vi "Auto Fit and Save Calibration Curve_YCC.vi"() -> ()   [LabVIEW 2014]
uses:
  <vilib>/Utility/file.llb/Write To Spreadsheet File (DBL).vi
  <vilib>/Utility/file.llb/Read From Spreadsheet File (DBL).vi
  <vilib>/Analysis/NI_AALPro.lvlib
  <vilib>/gmath/NI_Gmath.lvlib
panel:
  in  "defalut save?":bool=TRUE
  in  "X=T\nY=F":bool=TRUE
  out "save to path":path
  out "Polynomial Coefficients":dbl[](array[numeric])
  out "r^2":dbl format="%.7g"
  out "correlation coefficient r":dbl format="%.7g"
  out "folder exists?":bool
  in  "Save to Calibration File?":bool
  in  "Tab Control":enum32{"Sensitivity Fit", "Stiffness Fit"}(tab)
  in  "Folder Path":path
  out "Number of Files":i32
  in  "radius range wanted to fit (nm)":dbl=100.0
  out "All slope":dbl[](array[numeric])
  out "abs (All slope )":dbl[](array[numeric])
  out "XY Graph":cluster{dbl[], "abs (All slope )":dbl[]}[](graph)
  out "All laserpower (mW)":dbl[](array[numeric])
  out "Path":path
  in  "match substring":string="-Stuckbead Scan-"
  out "XY Graph 2":cluster{"all rows":dbl[], "all rows":dbl[]}[](graph)
  in  "file path (dialog if empty)":path
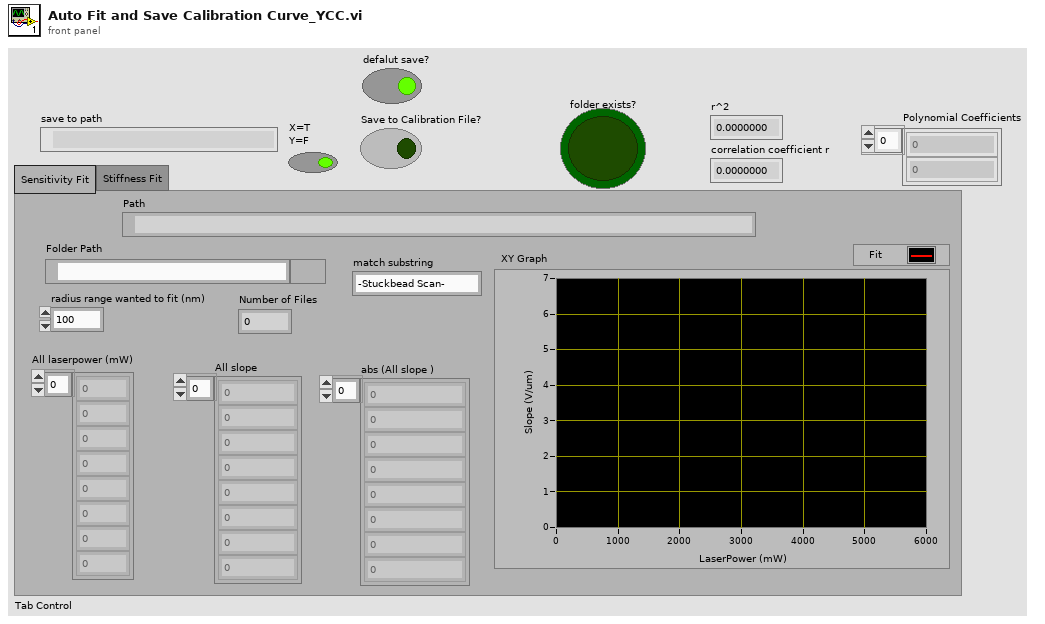
[diagram p1: front panel]
types:
  T1 = cluster{"All laserpower (mW)":dbl[], "Best Polynomial Fit":dbl[]}
  T2 = cluster{"All laserpower (mW)":dbl[], "abs (All slope )":dbl[]}
  T3 = cluster{"All laserpower (mW)":dbl[], "abs (All slope )":dbl[]}[]
  T4 = cluster{"all rows":dbl[], "Best Polynomial Fit":dbl[]}
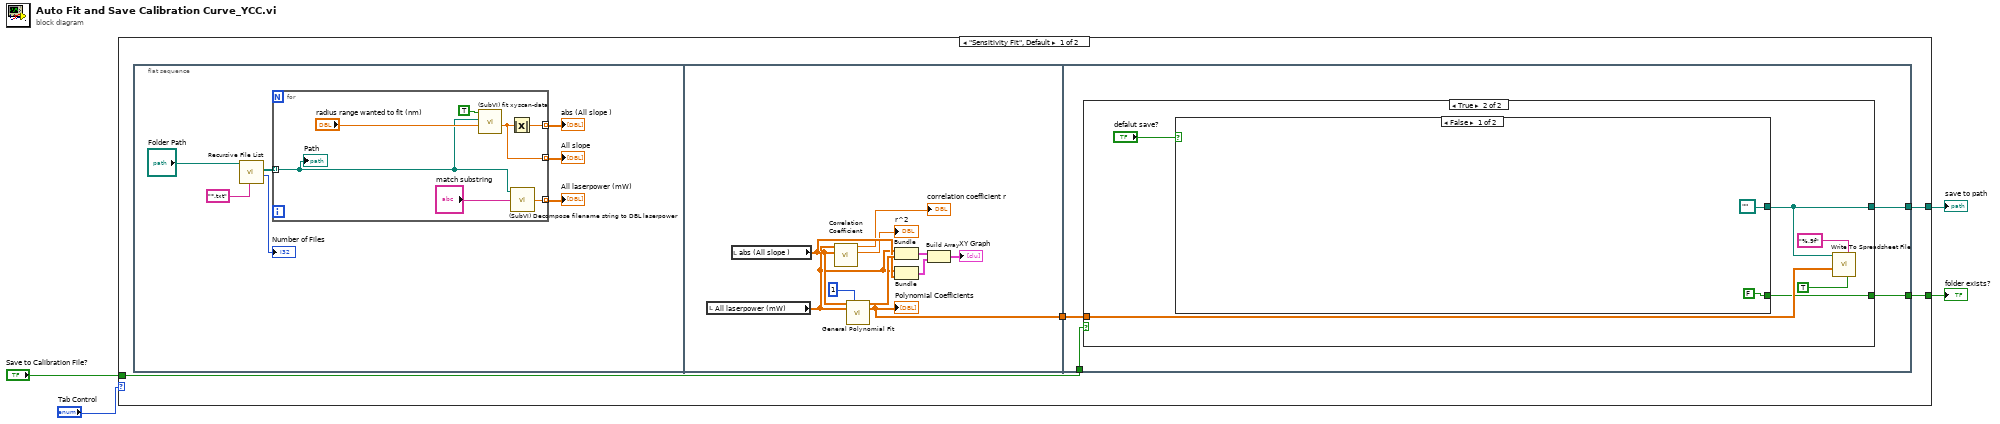
[diagram p0: block diagram]
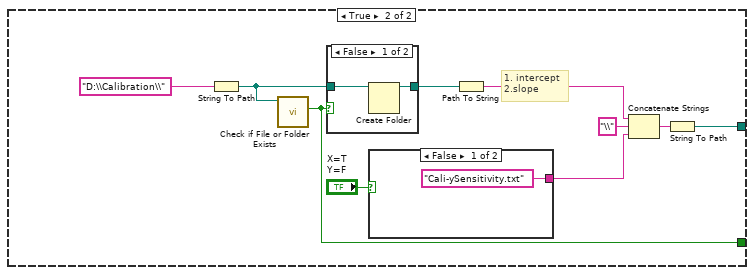
[diagram p3: hidden frame]
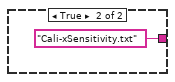
[diagram p4: hidden frame]
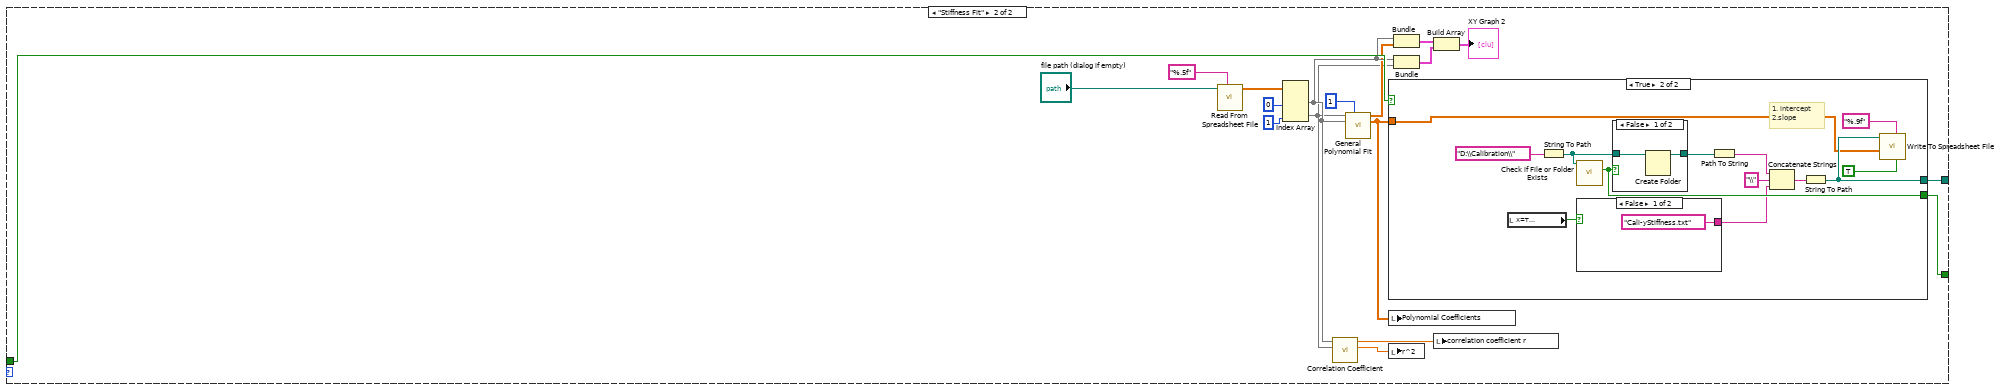
[diagram p6: hidden frame]
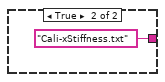
[diagram p8: hidden frame]
diagram:
  n1 = case shown="\"Sensitivity Fit\", Default" "Tab Control" {
    tunnel: "Save to Calibration File?" -> [w7 w77]
    tunnel: [w6 w75] -> w2
    tunnel: [w5 w76] -> w1
    frame "Sensitivity Fit", Default {
      n2 = flat-sequence {
        tunnel: [w24] -> w8
        tunnel: w8 -> [w36]
        tunnel: w7 -> [w35]
        tunnel: [w34] -> w6
        tunnel: [w33] -> w5
        frame #0 {
          n3 = call <vilib>:"Recursive File List.vi"("pattern"="*.txt", "Folder Path"="Folder Path") -> ("Number of Files"=→"Number of Files":i32, "All Files in Dir"=w12:path[])  [unwired: 5 in, 3 out]
          n4 = for {
            tunnel: w12 -> [w18] mode=indexing
            tunnel: [w20] -> w11 mode=indexing
            tunnel: [w19] -> w10 mode=indexing
            tunnel: [w17] -> w9 mode=indexing
            n5 = call "(SubVI) fit xyscan-data.vi"("range wanted to fit"="radius range wanted to fit (nm)", "file path (dialog if empty)"=w18, "X=T\nY=F"=TRUE ("X=T\nY=F")) -> ("Slope (V/um)"=w20:dbl)  [unwired: 4 in]
            n6 = Absolute Value(x=w20) -> (abs(x)=w19:dbl)
            n7 = call "(SubVI) Decompose filename string to DBL laserpower.vi"("match substring"="match substring", "path"=w18) -> ("LaserPower (mW)"=w17:dbl)  [unwired: 3 in]
            "Path" <- w18
          }
          "All slope" <- w11
          "abs (All slope )" <- w10
          "All laserpower (mW)" <- w9
        }
        frame #1 {
          n8 = local read "All laserpower (mW)"() -> (w23:dbl[])
          n9 = local read "abs (All slope )"() -> (w27:dbl[])
          n10 = call <vilib>:"Correlation Coefficient.vi"("Y"=w27, "X"=w23) -> ("r^2"=→"r^2":dbl, "correlation coefficient r"=→"correlation coefficient r":dbl)  [unwired: 8 in]
          n11 = call <vilib>:"General Polynomial Fit.vi"("Y"=w27, "polynomial order"=1, "X"=w23) -> ("Best Polynomial Fit"=w32:dbl[], "Polynomial Coefficients"=w24:dbl[])  [unwired: 9 in, 2 out]
          "Polynomial Coefficients" <- w24
          n12 = Bundle("All laserpower (mW)"=w23, "Best Polynomial Fit"=w32) -> (w31:T1)  [unwired: 1 in]
          n13 = Bundle("All laserpower (mW)"=w23, "abs (All slope )"=w27) -> (w30:T2)  [unwired: 1 in]
          n14 = Build Array(w31, w30) -> (→"XY Graph":T3)
        }
        frame #2 {
          n15 = case shown="True" w35 {
            tunnel: w36 -> [_ w42]
            tunnel: [_ w39] -> w34
            tunnel: [_ w38] -> w33
            frame False {
            }
            frame True {
              n16 = case shown="False" "defalut save?" {
                tunnel: [path "" w47] -> w39
                tunnel: [FALSE ("file or folder exists?") w46] -> w38
                frame False {
                }
                frame True {
                  # "1. intercept\n2.slope"
                  n17 = String To Path(string="D:\\Calibration\\") -> (path=w54:path)
                  n18 = call <vilib>:"Check if File or Folder Exists.vi"("path"=w54) -> ("file or folder exists?"=w46:bool)  [unwired: 8 in, 2 out]
                  n19 = case shown="False" w46 {
                    tunnel: w54 -> [w58 w59]
                    tunnel: [w57 w59] -> w52
                    frame False {
                      n20 = Create Folder(path (use dialog)=w58) -> (created path=w57:path)  [unwired: 2 in, 2 out]
                    }
                    frame True {
                    }
                  }
                  n21 = case shown="False" "X=T\nY=F" {
                    tunnel: ["Cali-ySensitivity.txt" "Cali-xSensitivity.txt"] -> w49
                    frame False {
                    }
                    frame True {
                    }
                  }
                  n22 = Path To String(path=w52) -> (string=w51:string)
                  n23 = Concatenate Strings(w51, "\\", w49) -> (w50:string)
                  n24 = String To Path(string=w50) -> (path=w47:path)
                }
              }
              n25 = call-poly <vilib>:"Write To Spreadsheet File.vi"("transpose? (no:F)"=TRUE, "format (%.3f)"="%.9f", "1D data"=w42, "file path (dialog if empty)"=w39) -> ()  [unwired: 4 in, 1 out]
            }
          }
        }
      }
    }
    frame "Stiffness Fit" {
      n26 = call-poly <vilib>:"Read From Spreadsheet File.vi"("format (%.3f)"="%.5f", "file path (dialog if empty)"="file path (dialog if empty)") -> ("all rows"=w72:dbl[][])  [unwired: 5 in, 4 out]
      n27 = Index Array(array=w72, index (col) #1=0 ("disabled index (col)"), index (col) #2=1 ("disabled index (col)")) -> (element #1=w64:dbl[], element #2=w62:dbl[])  [unwired: 2 in]
      n28 = call <vilib>:"Correlation Coefficient.vi"("Y"=w62, "X"=w64) -> ("r^2"=w67:dbl, "correlation coefficient r"=w68:dbl)  [unwired: 8 in]
      n29 = call <vilib>:"General Polynomial Fit.vi"("Y"=w62, "polynomial order"=1, "X"=w64) -> ("Best Polynomial Fit"=w63:dbl[], "Polynomial Coefficients"=w60:dbl[])  [unwired: 9 in, 2 out]
      n30 = case shown="True" w77 {
        tunnel: [_ w82] -> w76
        tunnel: [_ w81] -> w75
        tunnel: w60 -> [_ w80]
        frame False {
        }
        frame True {
          # "1. intercept\n2.slope"
          n31 = local read "X=T\nY=F"() -> (w79:bool)
          n32 = String To Path(string="D:\\Calibration\\") -> (path=w90:path)
          n33 = call <vilib>:"Check if File or Folder Exists.vi"("path"=w90) -> ("file or folder exists?"=w82:bool)  [unwired: 8 in, 2 out]
          n34 = case shown="False" w79 {
            tunnel: ["Cali-yStiffness.txt" "Cali-xStiffness.txt"] -> w78
            frame False {
            }
            frame True {
            }
          }
          n35 = case shown="False" w82 {
            tunnel: w90 -> [w94 w95]
            tunnel: [w93 w95] -> w88
            frame False {
              n36 = Create Folder(path (use dialog)=w94) -> (created path=w93:path)  [unwired: 2 in, 2 out]
            }
            frame True {
            }
          }
          n37 = Path To String(path=w88) -> (string=w87:string)
          n38 = Concatenate Strings(w87, "\\", w78) -> (w86:string)
          n39 = String To Path(string=w86) -> (path=w81:path)
          n40 = call-poly <vilib>:"Write To Spreadsheet File.vi"("transpose? (no:F)"=TRUE, "format (%.3f)"="%.9f", "1D data"=w80, "file path (dialog if empty)"=w81) -> ()  [unwired: 4 in, 1 out]
        }
      }
      n41 = local write "Polynomial Coefficients"(w60) -> ()
      n42 = local write "r^2"(w67) -> ()
      n43 = Bundle("all rows"=w64, "Best Polynomial Fit"=w63) -> (w66:T4)  [unwired: 1 in]
      n44 = Bundle("all rows"=w64, "all rows"=w62) -> (w65:cluster{"all rows":dbl[], "all rows":dbl[]})  [unwired: 1 in]
      n45 = Build Array(w66, w65) -> (→"XY Graph 2":cluster{"all rows":dbl[], "all rows":dbl[]}[])
      n46 = local write "correlation coefficient r"(w68) -> ()
    }
  }
  "folder exists?" <- w1
  "save to path" <- w2
